vi "Correct For FFT.vi"(8 "error in (no error)":errorcluster, 11 "Spectral Information in":dbl[](array[numeric])) -> (0 "error out":errorcluster, 3 "Spectral Information out":dbl[](array[numeric]))   [LabVIEW 2016]
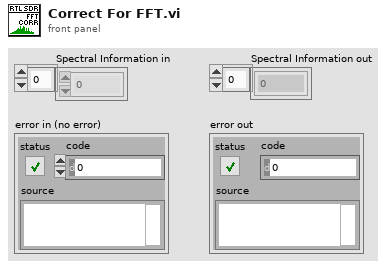
[diagram p1: front panel]
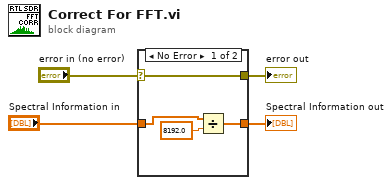
[diagram p0: block diagram]
diagram:
  n1 = case shown="No Error" "error in (no error)" {
    selector: "error in (no error)" -> [w6 w9]
    tunnel: "Spectral Information in" -> [w5 w10]
    tunnel: [w7 w10] -> w2
    tunnel: [w6 w9] -> w4
    frame No Error {
      n2 = Divide(x=w5, y=8192.0) -> (x/y=w7:dbl[])
    }
    frame Error {
    }
  }
  "error out" <- w4
  "Spectral Information out" <- w2
